vi "Data.Result Numeric Look Up Result Code.vi"(4 "Limits":variant, 6 "error in":errorcluster, 7 "Numeric":T1 {"Status" items=["LOG", "PASS", "FAIL", "ERROR"]}) -> (2 "Numeric Out":T1 {"Status" items=["LOG", "PASS", "FAIL", "ERROR"]})   [LabVIEW 2024, in "EQMF.lvlib" / "Data.lvlib"]
uses:
  Data.lvlib
  TypeDefs/Data.Result Numeric.ctl
  TypeDefs/Data.Result Numeric Limit Type.ctl
  TypeDefs/Data.Result Item Status.ctl
  TypeDefs/Data.Result Limit Definition.ctl
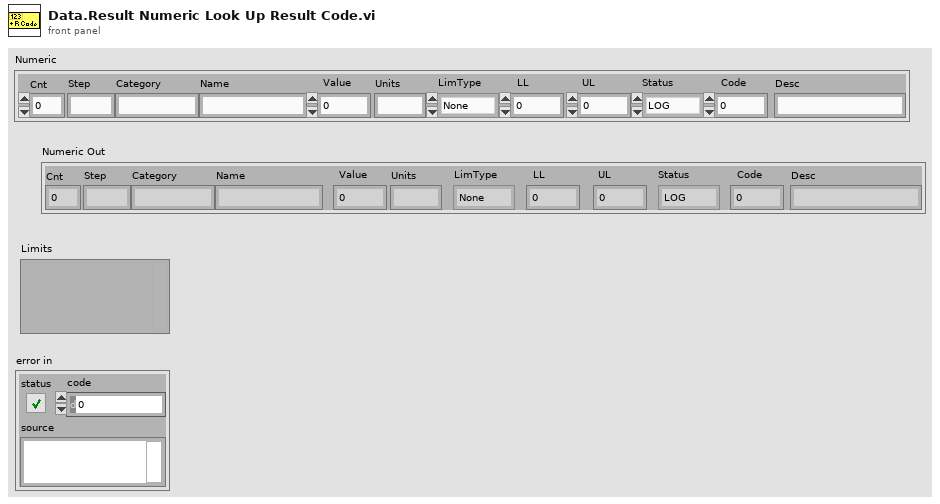
[diagram p1: front panel]
types:
  T1 = typedef "EQMF.lvlib/Data.lvlib/Data.Result Numeric.ctl" = cluster{"Cnt":i32, "Step":string, "Category":string, "Name":string, "Value":dbl, "Units":string, "LimType":T2, "LL":dbl, "UL":dbl, "Status":T3, "Code":i32, "Desc":string}
  T2 = typedef "EQMF.lvlib/Data.lvlib/Data.Result Numeric Limit Type.ctl" = enum16{"None", "EQ", "NE", "GT", "LT", "GE", "LE", "GTLT", "GELE", "GELT", "GTLE", "LTGT", "LEGE", "LEGT", "LTGE"}
  T3 = typedef "EQMF.lvlib/Data.lvlib/Data.Result Item Status.ctl" = i32
  T4 = typedef "EQMF.lvlib/Data.lvlib/Data.Result Limit Definition.ctl" = cluster{"Name":string, "LimType":T2, "LL":dbl, "UL":dbl, "Units":string, "FailCode":i32, "FailDesc":string}
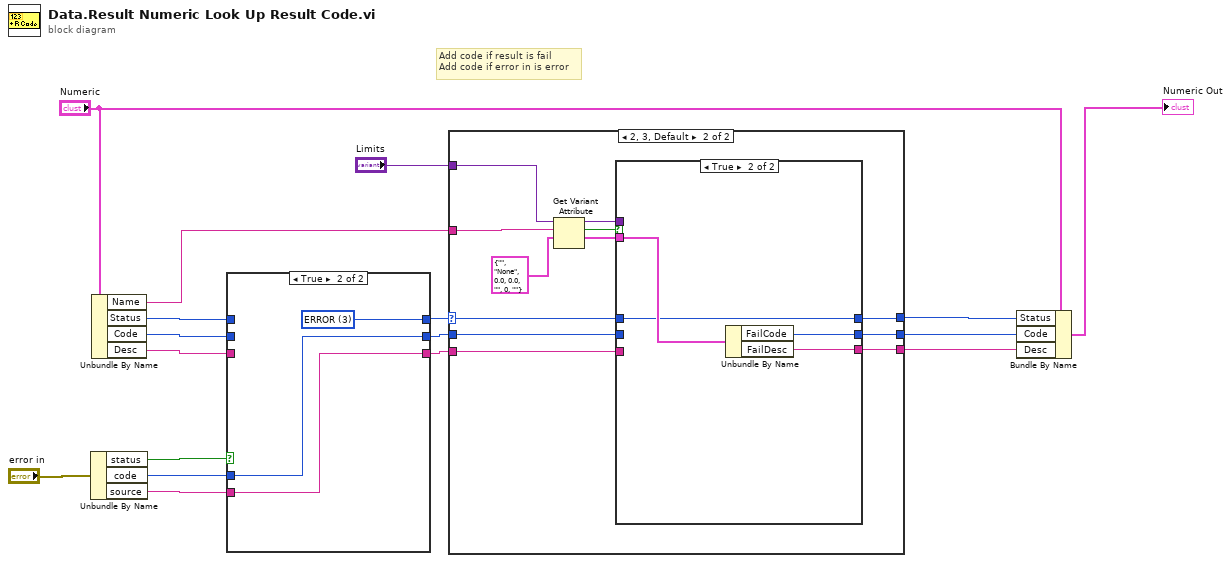
[diagram p0: block diagram]
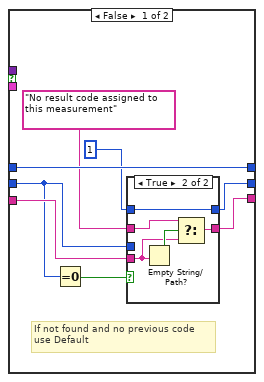
[diagram p3: hidden frame]
diagram:
  # "Add code if result is fail\nAdd code if error in is error"
  n1 = Unbundle By Name("error in") -> ("status"=w14:bool, "code"=w12:i32, "source"=w11:string)
  n2 = Unbundle By Name("Numeric") -> ("Name"=w5:string, "Status"=w13:T3, "Code"=w2:i32, "Desc"=w1:string)
  n3 = case shown="True" w14 {
    tunnel: [w20 w21] -> w10
    tunnel: w13 -> [w20 _]
    tunnel: w12 -> [_ w23]
    tunnel: [w19 w23] -> w8
    tunnel: w11 -> [_ w22]
    tunnel: [w18 w22] -> w7
    tunnel: w2 -> [w19 _]
    tunnel: w1 -> [w18 _]
    frame False {
    }
    frame True {
      w21 = T3 3 items=["LOG", "PASS", "FAIL", "ERROR"] ("Status")
    }
  }
  n4 = case shown="2, 3, Default" w10 {
    selector: w10 -> [w26 w30]
    tunnel: [w26 w29] -> w9
    tunnel: w8 -> [w25 w28]
    tunnel: w7 -> [w24 w27]
    tunnel: [w25 w33] -> w6
    tunnel: w5 -> [_ w34]
    tunnel: [w24 w32] -> w4
    tunnel: "Limits" -> [_ w31]
    frame 0, 1 {
      # "Log or PASS\nNo fail code"
    }
    frame 2, 3, Default {
      n5 = Get Variant Attribute(Variant=w31, name=w34, default value (empty Variant)=T4 {"Name"="", "LimType"=enum."None", "LL"=0.0, "UL"=0.0, "Units"="", "FailCode"=0, "FailDesc"=""} ("KATE_Lib.lvlib:Data.lvlib:Data.Result Limit Definition")) -> (duplicate Variant=w37:variant, found=w38:bool, value=w36:T4)  [unwired: 1 in, 1 out]
      n6 = case shown="True" w38 {
        tunnel: w37 -> [_ _]
        tunnel: w36 -> [_ w56]
        tunnel: [w42 w57] -> w33
        tunnel: [w41 w55] -> w32
        tunnel: w30 -> [w46 w54]
        tunnel: [w46 w54] -> w29
        tunnel: w28 -> [w43 _]
        tunnel: w27 -> [w44 _]
        frame False {
          # "If not found and no previous code\nuse Default"
          n7 = Equal To 0?(x=w43) -> (x = 0?=w45:bool)
          n8 = case shown="True" w45 {
            tunnel: w44 -> [w47 w50]
            tunnel: w43 -> [w48 _]
            tunnel: 1 ("Code") -> [_ w53]
            tunnel: "No result code assigned to this measurement" ("Desc") -> [_ w49]
            tunnel: [w48 w53] -> w42
            tunnel: [w47 w52] -> w41
            frame False {
            }
            frame True {
              n9 = Empty String/Path?(string/path=w50) -> (empty?=w51:bool)
              n10 = Select(t=w49, s=w51, f=w50) -> (s? t:f=w52:string)
            }
          }
        }
        frame True {
          n11 = Unbundle By Name(w56) -> ("FailCode"=w57:i32, "FailDesc"=w55:string)
        }
      }
    }
  }
  n12 = Bundle By Name(cluster="Numeric", "Status"=w9, "Code"=w6, "Desc"=w4) -> (→"Numeric Out":T1)
